vi "FPGAstatus_Reference.vi"() -> ()   [LabVIEW 2013]
uses:
  RIG-SPECIFIC FILES/FPGA Refs/FPGA Ref.ctl
panel:
  in  "FGPA Ref":T1
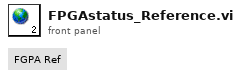
[diagram p1: front panel]
types:
  T1 = typedef "FPGA Ref.ctl" = refnum<k20>
diagram:
